vi "SQL表面型号数据库读取.vi"(8 "error in (no error)":errorcluster caption="错误输入（无错误）") -> (0 "error out":errorcluster caption="错误输出", 1 "已删除的部分":string[](array[string]), 2 "x > 0? 2":bool, 4 "元素":string)   [LabVIEW 2017]
panel:
  out "Data":string[][](array[string])
  out "子数组":string[](array[string])
  out "Type_c":string
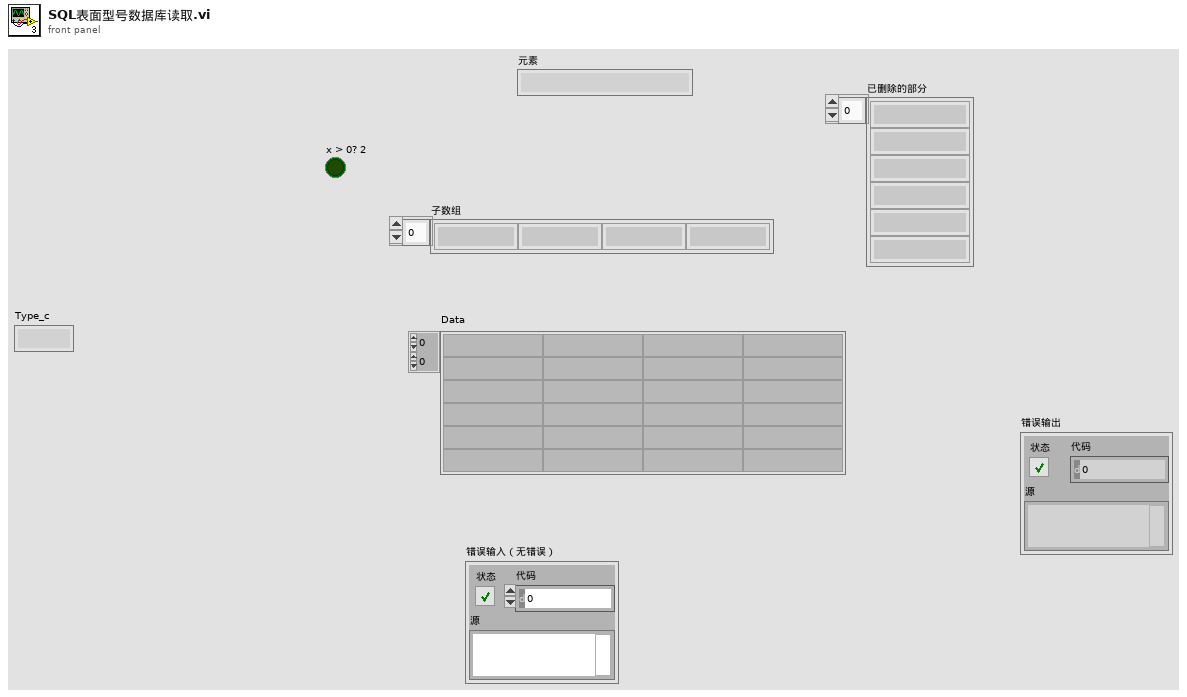
[diagram p1: front panel]
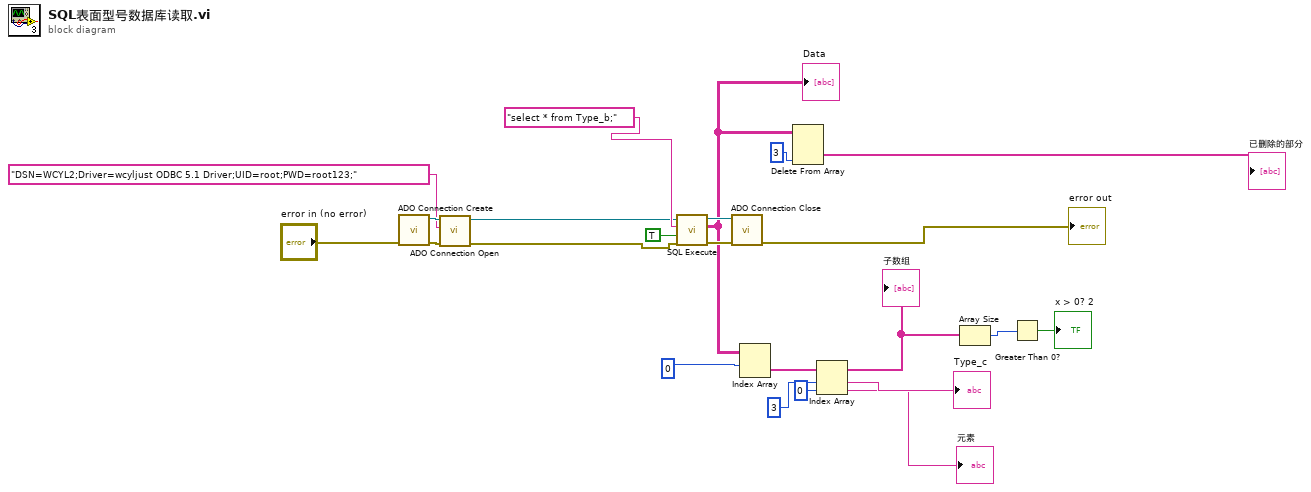
[diagram p0: block diagram]
diagram:
  n1 = call <userlib>:"ADO Connection Create.vi"("error in (no error)"="error in (no error)") -> ("error out"=w21:errorcluster, "ADODB._Connection Out"=w22:refnum<k7>)  [unwired: 9 in]
  n2 = call <userlib>:"ADO Connection Open.vi"("error in (no error)"=w21, "ConnectionString"="DSN=WCYL2;Driver=wcyljust ODBC 5.1 Driver;UID=root;PWD=root123;", "ADODB._Connection In"=w22) -> ("error out"=w1:errorcluster, "ADODB._Connection Out"=w2:refnum<k7>)  [unwired: 7 in]
  n3 = call <userlib>:"SQL Execute.vi"("error in (no error)"=w1, "Return Data (T)"=TRUE, "Command Text"="select * from Type_b;", "ADODB._Connection In"=w2) -> ("error out"=w14:errorcluster, "Data"=w8:string[][], "ADODB._Connection Out"=w15:refnum<k7>)  [unwired: 4 in, 1 out]
  "Data" <- w8
  n4 = call <userlib>:"ADO Connection Close.vi"("error in (no error)"=w14, "ADODB._Connection In"=w15) -> ("error out"=→"error out":errorcluster)  [unwired: 8 in, 1 out]
  n5 = Index Array(array=w8, index (row)=0 ("索引 (行)")) -> (element=w12:string[])  [unwired: 1 in]
  "子数组" <- w12
  n6 = Delete From Array(array=w8, index (col)=3 ("索引 (行)")) -> (deleted portion=→"已删除的部分":string[])  [unwired: 2 in, 1 out]
  n7 = Index Array(array=w12, index #1=3 ("索引"), index #2=0 ("索引")) -> (element #1=→"Type_c":string, element #2=→"元素":string)
  n8 = Array Size(array=w12) -> (size(s)=w11:i32)
  n9 = Greater Than 0?(x=w11) -> (x > 0?=→"x > 0? 2":bool)
